vi "Dialog.vi"(8 "error in (no error)":errorcluster, 10 "Settings In":T1) -> (0 "error out":errorcluster, 2 "Settings Out":T1)   [LabVIEW 2012]
panel:
  in  "Limit number of pages":dbl=3.0
  in  "Select Printer":string(combo)="Lab Printer 1"
  in  "Cancel Button":bool
  in  "OK Button":bool
  in  "Help":bool
  in  "When saving multiple files":enum32{"Radio Selection 1", "Radio Selection 2"}(radio)
  in  "Prompt for file path":bool
  in  "Filename":path
  # "Settings - Sine Wave Tester"
  # "Print Options"
  # "Save Options"
  # "When saving multiple files"
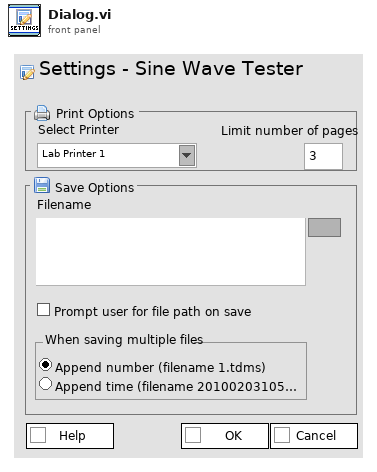
[diagram p1: front panel]
types:
  T1 = cluster{"Select Printer":string, "Limit number of pages":dbl, "Filename":path, "Prompt for file path":bool, "When saving multiple files":enum32{"Radio Selection 1", "Radio Selection 2"}}
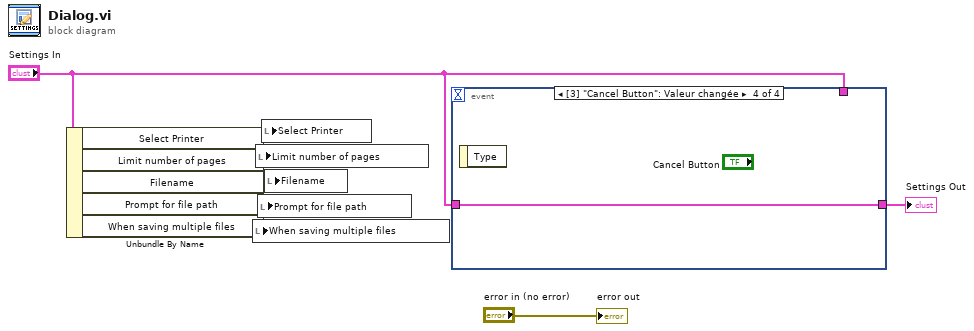
[diagram p0: block diagram]
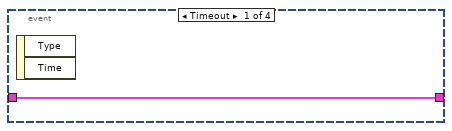
[diagram p2: hidden frame]
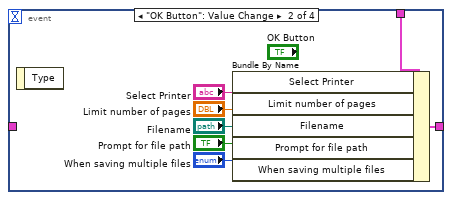
[diagram p3: hidden frame]
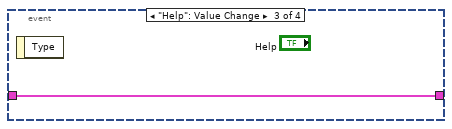
[diagram p4: hidden frame]
diagram:
  n1 = Unbundle By Name("Settings In") -> ("Select Printer"=w8:string, "Limit number of pages"=w7:dbl, "Filename"=w6:path, "Prompt for file path"=w5:bool, "When saving multiple files"=w4:enum32{"Radio Selection 1", "Radio Selection 2"})
  n2 = local write "When saving multiple files"(w4) -> ()
  n3 = local write "Limit number of pages"(w7) -> ()
  n4 = local write "Prompt for file path"(w5) -> ()
  n5 = local write "Select Printer"(w8) -> ()
  n6 = local write "Filename"(w6) -> ()
  n7 = event shown="[3] \"Cancel Button\": Valeur changée" {
    selector: _ -> [_ _ _ _]
    dyn-events: _ -> [_ _ _ _]
    timeout: _ -> [_ _ _ _]
    tunnel: "Settings In" -> [_ w16 _ _]
    tunnel: [w9 w10 w17 w18] -> w3
    tunnel: "Settings In" -> [w9 _ w17 w18]
    event Timeout {
      n8 = event-data() -> ()  [unwired: 1 in, 2 out]
    }
    event "OK Button": Value Change {
      n9 = event-data() -> ()  [unwired: 1 in, 1 out]
      n10 = Bundle By Name(cluster=w16, "Select Printer"="Select Printer", "Limit number of pages"="Limit number of pages", "Filename"="Filename", "Prompt for file path"="Prompt for file path", "When saving multiple files"="When saving multiple files") -> (w10:T1)
    }
    event "Help": Value Change {
      n11 = event-data() -> ()  [unwired: 1 in, 1 out]
    }
    event "Cancel Button": Value Change {
      n12 = event-data() -> ()  [unwired: 1 in, 1 out]
    }
  }
  "Settings Out" <- w3
  "error out" <- "error in (no error)"
